vi "CompareTwoValues.vi"(1 "number2":dbl, 2 "number1":dbl) -> (0 "x < y?":bool)   [LabVIEW 2014, in "Panels.lvlib"]
uses:
  Panels.lvlib
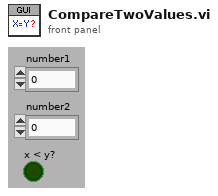
[diagram p1: front panel]
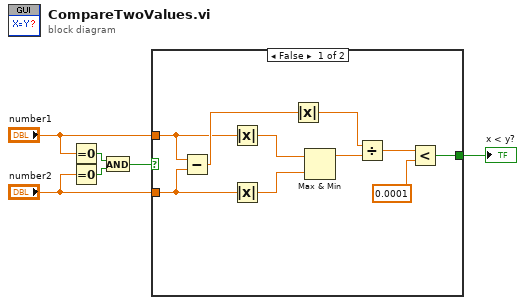
[diagram p0: block diagram]
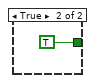
[diagram p2: hidden frame]
diagram:
  n1 = Equal To 0?(x="number1") -> (x = 0?=w2:bool)
  n2 = Equal To 0?(x="number2") -> (x = 0?=w3:bool)
  n3 = And(x=w2, y=w3) -> (x .and. y?=w1:bool)
  n4 = case shown="False" w1 {
    tunnel: [w10 TRUE] -> w6
    tunnel: "number1" -> [w9 _]
    tunnel: "number2" -> [w8 _]
    frame False {
      n5 = Subtract(x=w9, y=w8) -> (x-y=w13:dbl)
      n6 = Absolute Value(x=w9) -> (abs(x)=w16:dbl)
      n7 = Absolute Value(x=w8) -> (abs(x)=w15:dbl)
      n8 = Absolute Value(x=w13) -> (abs(x)=w7:dbl)
      n9 = Max & Min(x=w16, y=w15) -> (max(x,y)=w14:dbl)  [unwired: 1 out]
      n10 = Divide(x=w7, y=w14) -> (x/y=w12:dbl)
      n11 = Less?(x=w12, y=0.0001) -> (x < y?=w10:bool)
    }
    frame True {
    }
  }
  "x < y?" <- w6
